vi "curv avg.vi"(0 "curv avg array in":dbl[][][](array[numeric]), 2 "5 col curv":dbl[][](array[numeric])=[[3.0, 3.0, 3.0, 3.0, 3.0]], 4 "sen plt num":i32) -> (14 "curv avg array out":dbl[][][](array[numeric]))   [LabVIEW 2019]
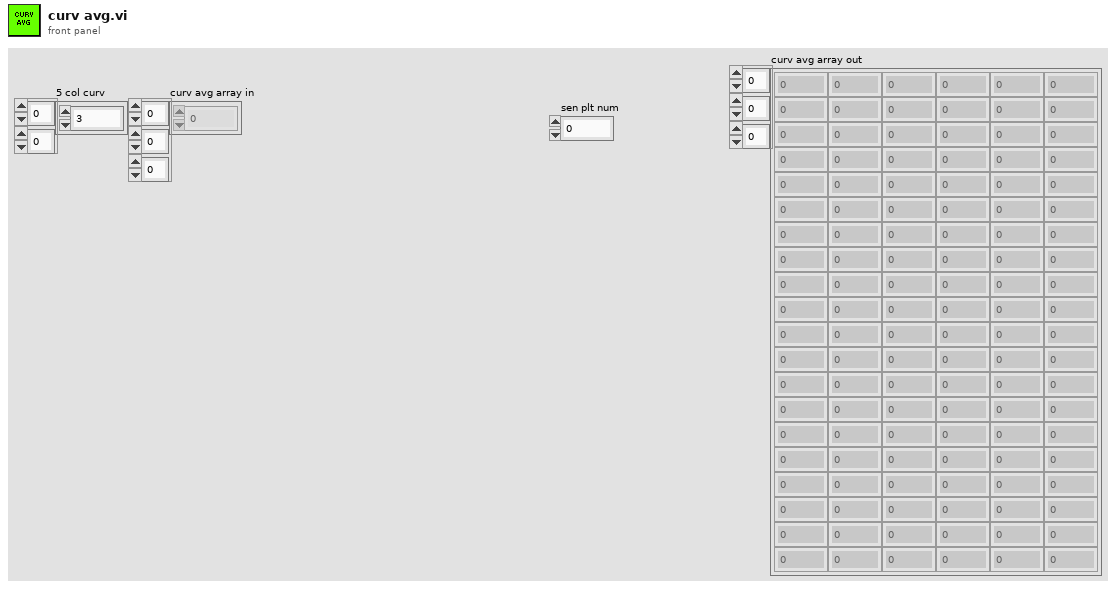
[diagram p1: front panel]
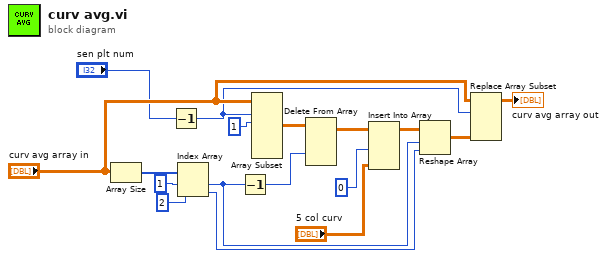
[diagram p0: block diagram]
diagram:
  n1 = Array Size(array="curv avg array in") -> (size(s)=w13:i32[])
  n2 = Decrement(x="sen plt num") -> (x-1=w6:i32)
  n3 = Index Array(array=w13, index #1=1 ("index"), index #2=2 ("index")) -> (element #1=w2:i32, element #2=w3:i32)
  n4 = Decrement(x=w2) -> (x-1=w11:i32)
  n5 = Array Subset(array="curv avg array in", index (dim 0)=w6, length (dim 0)=1 ("length")) -> (w16:dbl[][][])  [unwired: 4 in]
  n6 = Delete From Array(array=w16, index (dim 1)=w11) -> (array with subset deleted=w15:dbl[][][])  [unwired: 3 in, 1 out]
  n7 = Insert Into Array(array=w15, index (dim 1)=0 ("disabled index (row)"), new element="5 col curv") -> (w10:dbl[][][])  [unwired: 2 in]
  n8 = Reshape Array(w10, w2, w3) -> (w9:dbl[][])
  n9 = Replace Array Subset(array="curv avg array in", new element=w9, index (dim 0)=w6) -> (→"curv avg array out":dbl[][][])  [unwired: 2 in]
